vi "N分之一的数列和.vi"(11 "Num":i32=100) -> (3 "Result":dbl)   [LabVIEW 2012]
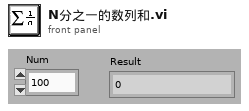
[diagram p1: front panel]
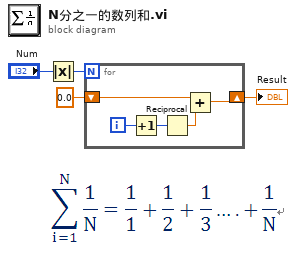
[diagram p0: block diagram]
diagram:
  n1 = Absolute Value(x="Num") -> (abs(x)=w3:i32)
  n2 = for {
    N: w3 -> [_]
    shift-right: [w7] -> w1
    shift-left: 0.0 -> [w8]
    i -> [w6]
    n3 = Increment(x=w6) -> (x+1=w5:i32)
    n4 = Reciprocal(x=w5) -> (1/x=w9:dbl)
    n5 = Add(x=w8, y=w9) -> (x+y=w7:dbl)
  }
  "Result" <- w1
